vi "cmd_interface_test.vi"() -> ()   [LabVIEW 2013]
panel:
  out "result":dbl format="%#_13g"
  out "数组":dbl[](array[numeric])
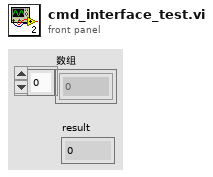
[diagram p1: front panel]
types:
  T1 = cluster{"cmd":refnum<user-event>, "cmd":cluster{"cmd":string, "value":dbl, "result ":refnum<vi>, "channel":i32, "on/off":bool}}
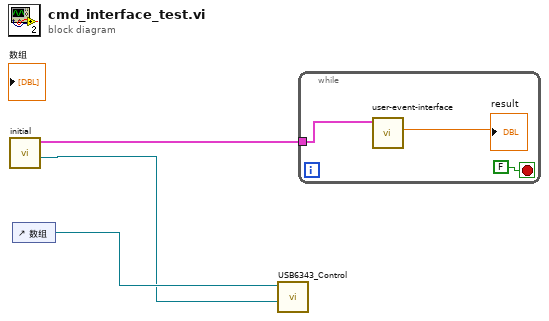
[diagram p0: block diagram]
diagram:
  n1 = call "initial.vi"() -> ("event rsg handle"=w1:refnum<event-registration>, "msg interface"=w2:T1)  [unwired: 10 in]
  n2 = control-ref of="数组"() -> (w3:refnum<vi>)
  n3 = call "USB6343_Control.vi"("event rsg handle"=w1, "monitor buff"=w3) -> ()  [unwired: 9 in, 1 out]
  n4 = while {
    tunnel: w2 -> [w4]
    stop <- FALSE stop-if-true
    n5 = call "user-event-interface.vi"("msg interface"=w4) -> ("result"=→"result":dbl)  [unwired: 9 in, 1 out]
  }
